vi "WMP Play File Simple.vi"() -> ()   [LabVIEW 2018, in "WMP.lvclass"]
uses:
  WMP.lvclass
panel:
  in  "Timeout [ms] (10000)":u32=10000
  in  "Sound File Path":path
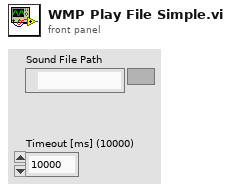
[diagram p1: front panel]
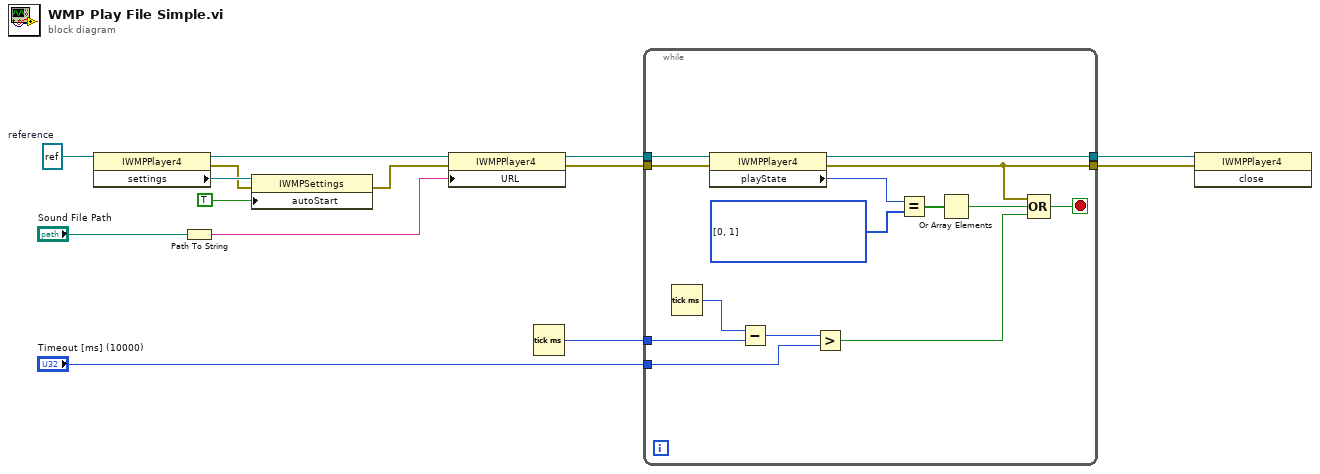
[diagram p0: block diagram]
diagram:
  w8 = refnum<k7> refnum  # reference
  n1 = property class="IWMPPlayer4"(reference=w8) -> (reference out=w10:refnum<k7>, error out=w11:errorcluster, "settings"=w13:refnum<k7>)  [unwired: 1 in]
  n2 = Path To String(path="Sound File Path") -> (string=w14:string)
  n3 = property class="IWMPSettings"(reference=w13, error in=w11, "autoStart"=TRUE) -> (error out=w9:errorcluster)  [unwired: 1 out]
  n4 = property class="IWMPPlayer4"(reference=w10, error in=w9, "URL"=w14) -> (reference out=w6:refnum<k7>, error out=w5:errorcluster)
  n5 = Tick Count (ms)() -> (millisecond timer value=w3:u32)
  n6 = while {
    tunnel: w6 -> [w28]
    tunnel: w5 -> [w27]
    tunnel: "Timeout [ms] (10000)" -> [w20]
    tunnel: w3 -> [w22]
    tunnel: [w16] -> w2
    tunnel: [w15] -> w1
    stop <- w17 stop-if-true
    w25 = i32[] [0, 1] items=["wmppsUndefined", "wmppsStopped", "wmppsPaused", "wmppsPlaying", "wmppsScanForward", "wmppsScanReverse", "wmppsBuffering", "wmppsWaiting", "wmppsMediaEnded", "wmppsTransitioning", "wmppsReady", "wmppsReconnecting", "wmppsLast"]
    n7 = Tick Count (ms)() -> (millisecond timer value=w23:u32)
    n8 = property class="IWMPPlayer4"(reference=w28, error in=w27) -> (reference out=w16:refnum<k7>, error out=w15:errorcluster, "playState"=w26:i32)
    n9 = Subtract(x=w23, y=w22) -> (x-y=w21:u32)
    n10 = Greater?(x=w21, y=w20) -> (0:w19:bool)
    n11 = Equal?(x=w26, y=w25) -> (x = y?=w24:bool[])
    n12 = Or Array Elements(Boolean array=w24) -> (logical OR=w18:bool)
    n13 = Compound Arithmetic op=OR(w15, w18, w19) -> (w17:bool)
  }
  n14 = invoke class="IWMPPlayer4" method="close"(reference=w2, error in=w1) -> ()  [unwired: 1 in, 3 out]
